vi "Do Async Auth.vi"(6 "Failed Response":refnum<class "Response.lvclass">, 7 "Complete Response":refnum<class "Response.lvclass">, 8 "error in (no error)":errorcluster, 9 "Timeout S (60)":dbl=60.0, 10 "Authorization in (New)":refnum<class "Authorization.lvclass">, 11 "OAuth2 in":refnum<class "OAuth2.lvclass">) -> (0 "error out":errorcluster, 1 "Async Authentication":refnum<class "Async Authorization.lvclass">, 3 "OAuth2 out":refnum<class "OAuth2.lvclass">)   [LabVIEW 2020, in "OAuth2.lvlib" / "OAuth2.lvclass"]
uses:
  OAuth2.lvclass
  Authorization/Authorization.lvclass
  Async Authorization/Async Authorization.lvclass
  Auth Async.vi
  OAuth2.lvclass/OAuth2.ctl
  HTTP Utils/Response/Response.lvclass
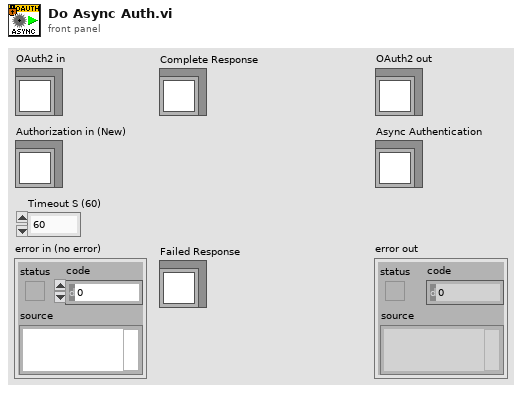
[diagram p1: front panel]
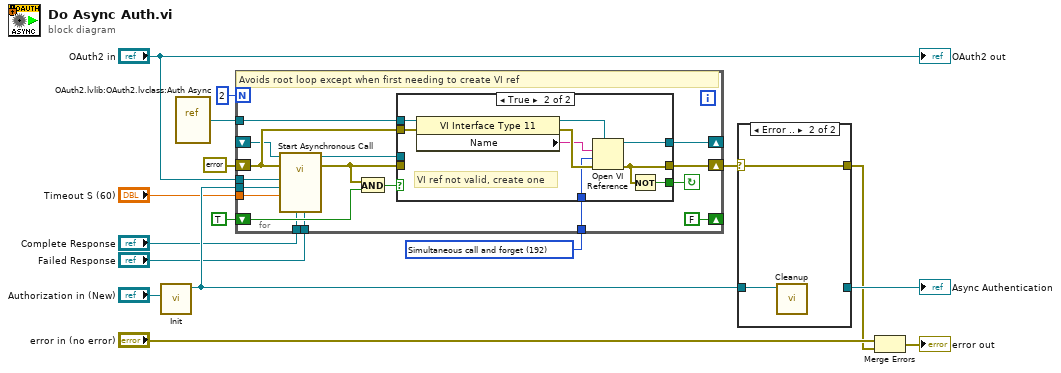
[diagram p0: block diagram]
diagram:
  w13 = 192 items=["Record modifications"=1, "Open templates for editing"=2, "Prompt user to save"=4, "Prepare for reentrant run"=8, "Prompt to find missing subVIs"=16, "Hide loading dialog box"=32, "Enable simultaneous calls"=64, "Prepare to call and forget"=128, "Simultaneous call and forget"=192, "Prepare to call and collect"=256, "Simultaneous call and collect"=320]
  n1 = call "Init.vi"("Authorization"="Authorization in (New)") -> ("Async Authorization out"=w7:refnum<class "Async Authorization.lvclass">)  [unwired: 9 in, 1 out]
  n2 = vi-ref "OAuth2.lvlib:OAuth2.lvclass:Auth Async.vi"() -> (w12:refnum<vi>)
  n3 = for {
    N: 2 -> [_]
    tunnel: w12 -> [w32]
    tunnel: w13 -> [w31]
    shift-right: [w30] -> _
    shift-left: _ -> [w29]
    shift-right: [w27] -> w8
    shift-left: errorcluster {"status"=FALSE, "code"=0, "source"=""} ("error constant") -> [w33]
    shift-right: [FALSE] -> _
    shift-left: TRUE -> [w24]
    tunnel: "OAuth2 in" -> [w21]
    tunnel: w7 -> [w20]
    tunnel: "Timeout S (60)" -> [w19]
    tunnel: "Complete Response" -> [w18]
    tunnel: "Failed Response" -> [w17]
    stop <- w23 continue-if-true
    # "Avoids root loop except when first needing to create VI ref"
    n4 = call-by-ref "Start Asynchronous Call"(reference=w29, error in=w33, "Failed Response"=w17, "Complete Response"=w18, "Timeout S"=w19, "Async Authorization"=w20, "OAuth2 in"=w21) -> (reference out=w28:refnum<vi>, error out=w26:errorcluster)  [unwired: 7 in]
    n5 = And(x=w26, y=w24) -> (x .and. y?=w25:bool)
    n6 = case shown="True" w25 {
      tunnel: w32 -> [_ w43]
      tunnel: w31 -> [_ w41]
      tunnel: [w35 w39] -> w30
      tunnel: w28 -> [w35 _]
      tunnel: [w34 w37] -> w27
      tunnel: w26 -> [w34 _]
      tunnel: w33 -> [_ w38]
      tunnel: [_ w36] -> w23
      frame False {
        # "Keep reusing valid VI ref"
      }
      frame True {
        # "VI ref not valid, create one"
        n7 = property class="VI Interface Type 11"(reference=w43, error in=w38) -> (reference out=w40:refnum<vi>, error out=w44:errorcluster, "Name"=w42:string)
        n8 = Open VI Reference(type specifier VI Refnum (for type only)=w40, vi path=w42, options=w41, error in (no error)=w44) -> (vi reference=w39:refnum<vi>, error out=w37:errorcluster)  [unwired: 2 in]
        n9 = Not(x=w37) -> (.not. x?=w36:bool)
      }
    }
  }
  n10 = case shown="Error .." w8 {
    selector: w8 -> [_ w46]
    tunnel: w7 -> [w45 w47]
    tunnel: [w45 _] -> w6
    tunnel: [_ w46] -> w4
    frame No Error {
    }
    frame Error {
      n11 = call "Cleanup.vi"("Async Authorization in"=w47) -> ()  [unwired: 10 in, 1 out]
    }
  }
  "Async Authentication" <- w6
  n12 = Merge Errors("error in (no error)", w4) -> (→"error out":errorcluster)
  "OAuth2 out" <- "OAuth2 in"
